vi "Close Reference.vi"(8 "error in (no error)":errorcluster, 11 "Item in":refnum<class "Item.lvclass">) -> (0 "error out":errorcluster, 3 "Item out":refnum<class "Item.lvclass">)   [LabVIEW 2020, in "Code Cleanup.lvlib" / "Item.lvclass"]
uses:
  Item.lvclass
  Item.lvclass/Item.ctl
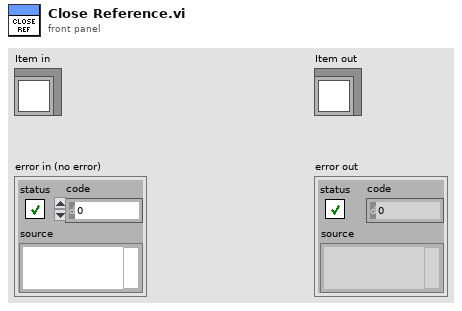
[diagram p1: front panel]
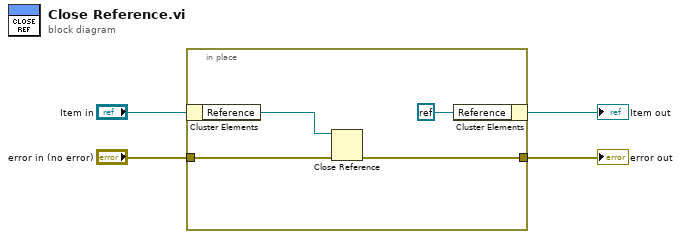
[diagram p0: block diagram]
diagram:
  n1 = in-place {
    in-place-border: "error in (no error)" -> [w8]
    in-place-border: [w7] -> w2
    n2 = in-place-cluster #1("Item in") -> ("Reference"=w6:refnum<vi>)
    n3 = Close Reference(reference=w6, error in (no error)=w8) -> (error out=w7:errorcluster)
    n4 = in-place-cluster #1("Reference"=refnum<k0> refnum) -> (→"Item out":refnum<class "Item.lvclass">)
  }
  "error out" <- w2
